vi "ElmoPosScale.vi"(1 "Elmo eCAT pos":i32) -> (0 "Elmo pos (rev)":dbl)   [LabVIEW 2018]
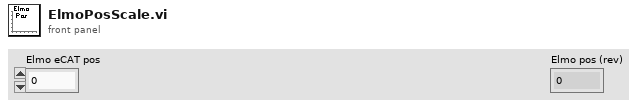
[diagram p1: front panel]
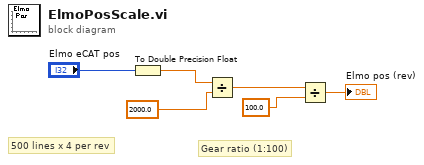
[diagram p0: block diagram]
diagram:
  # "500 lines x 4 per rev"
  # "Gear ratio (1:100)"
  n1 = To Double Precision Float(number="Elmo eCAT pos") -> (double precision float=w6:dbl)
  n2 = Divide(x=w6, y=2000.0) -> (x/y=w4:dbl)
  n3 = Divide(x=w4, y=100.0) -> (x/y=→"Elmo pos (rev)":dbl)
